vi "tarea avance.vi"() -> ()   [LabVIEW 2020]
panel:
  in  "Stop":bool
  out "Result":i32
  in  "Operate\nsubtract":bool
  in  "Operate\nplus":bool
  in  "Subtract":i32
  in  "Plus":i32
  # "Creado por Juan Andrés Bermúdez Gómez\nEstudiante de la Escuela de Aviación del Ejército\nPrograma de Ingeniería Aeronáutica"
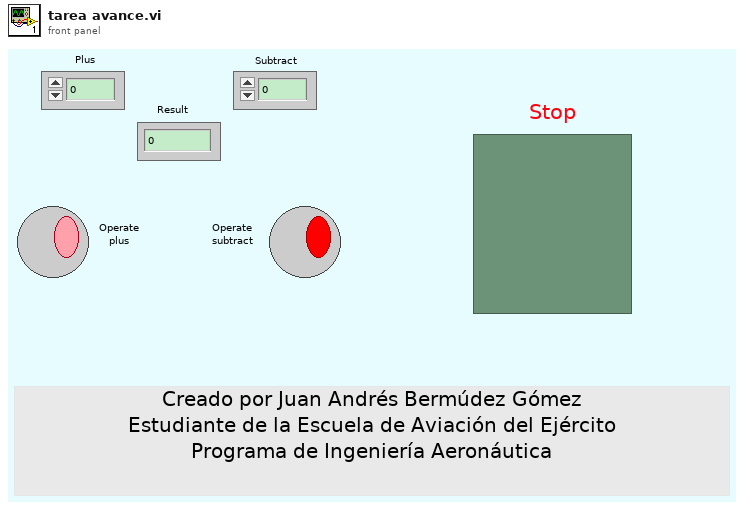
[diagram p1: front panel]
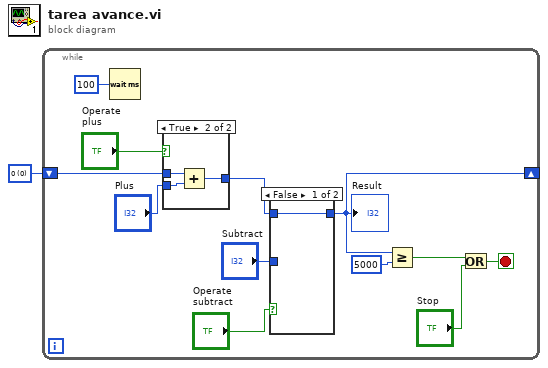
[diagram p0: block diagram]
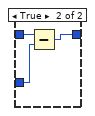
[diagram p2: hidden frame]
diagram:
  w1 = u16 0 items=["0"]
  n1 = while {
    shift-right: [w6] -> _
    shift-left: w1 -> [w8]
    stop <- w2 stop-if-true
    n2 = Wait (ms)(milliseconds to wait=100) -> ()  [unwired: 1 out]
    n3 = case shown="True" "Operate\nplus" {
      tunnel: "Plus" -> [_ w20]
      tunnel: w8 -> [w18 w21]
      tunnel: [w18 w19] -> w7
      frame False {
      }
      frame True {
        n4 = Add(x=w21, y=w20) -> (x+y=w19:i32)
      }
    }
    n5 = case shown="False" "Operate\nsubtract" {
      tunnel: "Subtract" -> [_ w17]
      tunnel: [w14 w16] -> w6
      tunnel: w7 -> [w14 w15]
      frame False {
      }
      frame True {
        n6 = Subtract(x=w15, y=w17) -> (x-y=w16:i32)
      }
    }
    "Result" <- w6
    n7 = Greater Or Equal?(x=w6, y=5000) -> (x >= y?=w4:bool)
    n8 = Or(x=w4, y="Stop") -> (x .or. y?=w2:bool)
  }
